vi "Box IDs Common Characters.vi"(8 "Error In":errorcluster, 10 "Box in":string, 11 "Box 1":string) -> (0 "Error Out":errorcluster, 3 "Common Characters":string)   [LabVIEW 2019]
doc: "This VI follows \"Box IDs Differ by 1 Char\" - using both Box IDs, find the mismatch index in order to return the common characters between the two Box IDs."
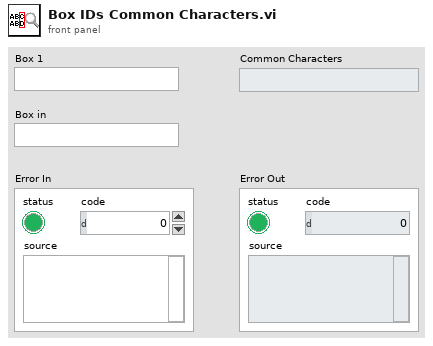
[diagram p1: front panel]
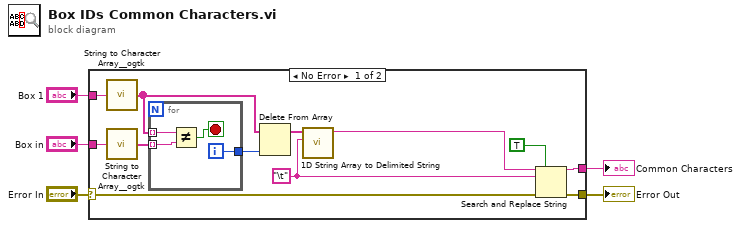
[diagram p0: block diagram]
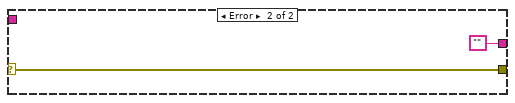
[diagram p2: hidden frame]
diagram:
  n1 = case shown="No Error" "Error In" {
    selector: "Error In" -> [w7 w22]
    tunnel: [w9 ""] -> w5
    tunnel: "Box in" -> [w13 _]
    tunnel: "Box 1" -> [w12 _]
    tunnel: [w6 w22] -> w1
    frame No Error {
      w10 = "\t"
      n2 = call <userlib>:"String to Character Array__ogtk.vi"("Input String"=w12) -> ("Character Array"=w14:string[])
      n3 = call <userlib>:"String to Character Array__ogtk.vi"("Input String"=w13) -> ("Character Array"=w15:string[])
      n4 = for {
        tunnel: w14 -> [w21] mode=indexing
        tunnel: w15 -> [w20] mode=indexing
        tunnel: [w18] -> w16
        i -> [w18]
        stop <- w19 stop-if-true
        n5 = Not Equal?(x=w21, y=w20) -> (x != y?=w19:bool)
      }
      n6 = Delete From Array(array=w14, index=w16) -> (array with subset deleted=w17:string[])  [unwired: 1 in, 1 out]
      n7 = call <vilib>:"1D String Array to Delimited String.vi"("delimiter"=w10, "string array"=w17) -> ("delimited string"=w11:string)  [unwired: 9 in]
      n8 = Search and Replace String(replace all?=TRUE ("replace all? (F)"), input string=w11, search string=w10, error in=w7) -> (result string=w9:string, error out=w6:errorcluster)  [unwired: 4 in, 2 out]
    }
    frame Error {
    }
  }
  "Common Characters" <- w5
  "Error Out" <- w1
